vi "Resistance to Colors.vi"() -> ()   [LabVIEW 2014]
panel:
  in  "Resistance Measured 2":dbl=46600.0
  out "Resistance Measured":dbl=46600.0
  out "Band 3":u32(colorbox)=16750592
  out "Band 2":u32(colorbox)=16067327
  out "Band 1":u32(colorbox)=16776960
  in  "Resistor Colors":u32[](array[colorbox])=[0, 16730368, 16711680, 16750592, 16776960, 6618880, 3381759, 16067327, 11776947, 16448250]
  # "0"
  # "1"
  # "2"
  # "3"
  # "4"
  # "5"
  # "6"
  # "7"
  # "8"
  # "9"
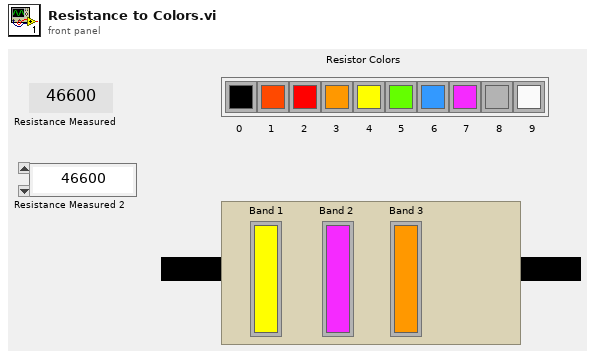
[diagram p1: front panel]
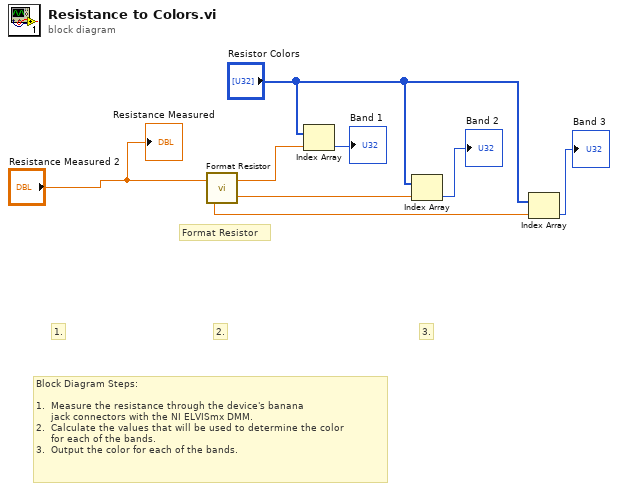
[diagram p0: block diagram]
diagram:
  # "Block Diagram Steps:\n\n1.  Measure the resistance through the device's banana\n     jack connectors with the NI ELVISmx DMM.\n2.  Calculate the values that will be used to determine the color\n     for each of the bands.\n3.  Output the color for each of the bands."
  # "2."
  # "3."
  # "1."
  # "Format Resistor"
  n1 = call "Format Resistor.vi"("Resistor Value"="Resistance Measured 2") -> ("Band 2"=w3:dbl, "Band 1"=w4:dbl, "Band3"=w2:dbl)
  n2 = Index Array(array="Resistor Colors", index=w4) -> (element=→"Band 1":u32)
  n3 = Index Array(array="Resistor Colors", index=w3) -> (element=→"Band 2":u32)
  n4 = Index Array(array="Resistor Colors", index=w2) -> (element=→"Band 3":u32)
  "Resistance Measured" <- "Resistance Measured 2"
